vi "Calibrate.vi"(0 "CART TCP Connection In":refnum<k5>, 7 "Calibrate Config":T1={"Frequency, MHz"=2412, "TX Gain"=0, "Data Rate"="1,0,0", "Packet Length"=4, "Packet Count"=4}, 11 "error in (no error)":errorcluster) -> (4 "CART TCP Connection Out":refnum<k5>, 6 "Messages Logged":string[](array[string]), 14 "Command Sent":string, 15 "error out":errorcluster)   [LabVIEW 2011, in "ART2 Test Panel.lvlib"]
uses:
  ART2 Test Panel.lvlib
  Controls/Calibrate Config.ctl
  CART/Controls/Data Rates.ctl
  Controls/Calibrate TXP modes.ctl
  CART/Controls/Inter Frame Spacing modes.ctl
  CART/Controls/Parameter.ctl
  SubVIs/NART Constants.vi
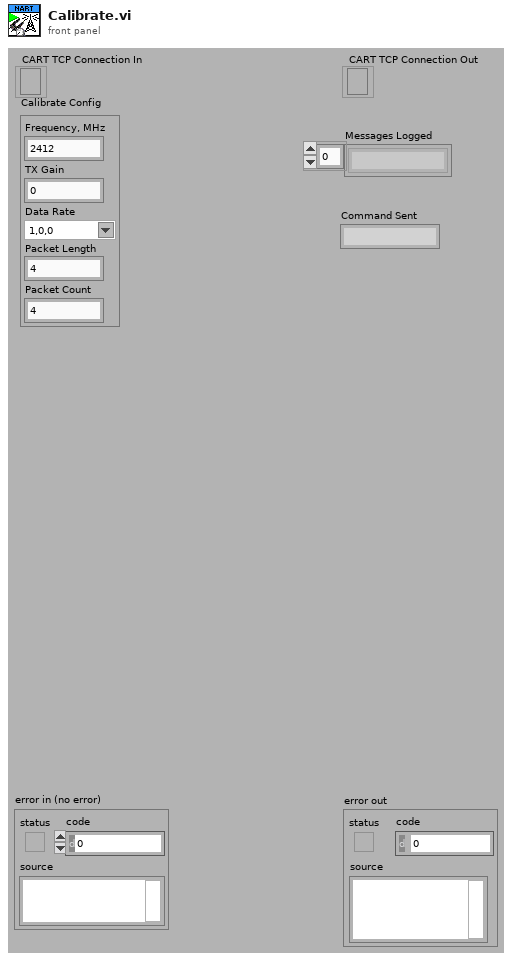
[diagram p1: front panel]
types:
  T1 = typedef "ART2 Test Panel.lvlib/Calibrate Config.ctl" = cluster{"Frequency, MHz":u32, "TX Gain":u32, "Data Rate":T2, "Packet Length":u32, "Packet Count":i32}
  T2 = typedef "ART2 Test Panel.lvlib/Data Rates.ctl" = string
  T3 = typedef "Calibrate TXP modes.ctl" = enum16{"none", "combined", "isolated", "iterate-combined ", "iterate-isolated"}
  T4 = typedef "ART2 Test Panel.lvlib/Parameter.ctl" = cluster{"Name":string, "Type":enum16{"decimal", "string", "float", "hex"}}
  T5 = typedef "ART2 Test Panel.lvlib/Inter Frame Spacing modes.ctl" = i16
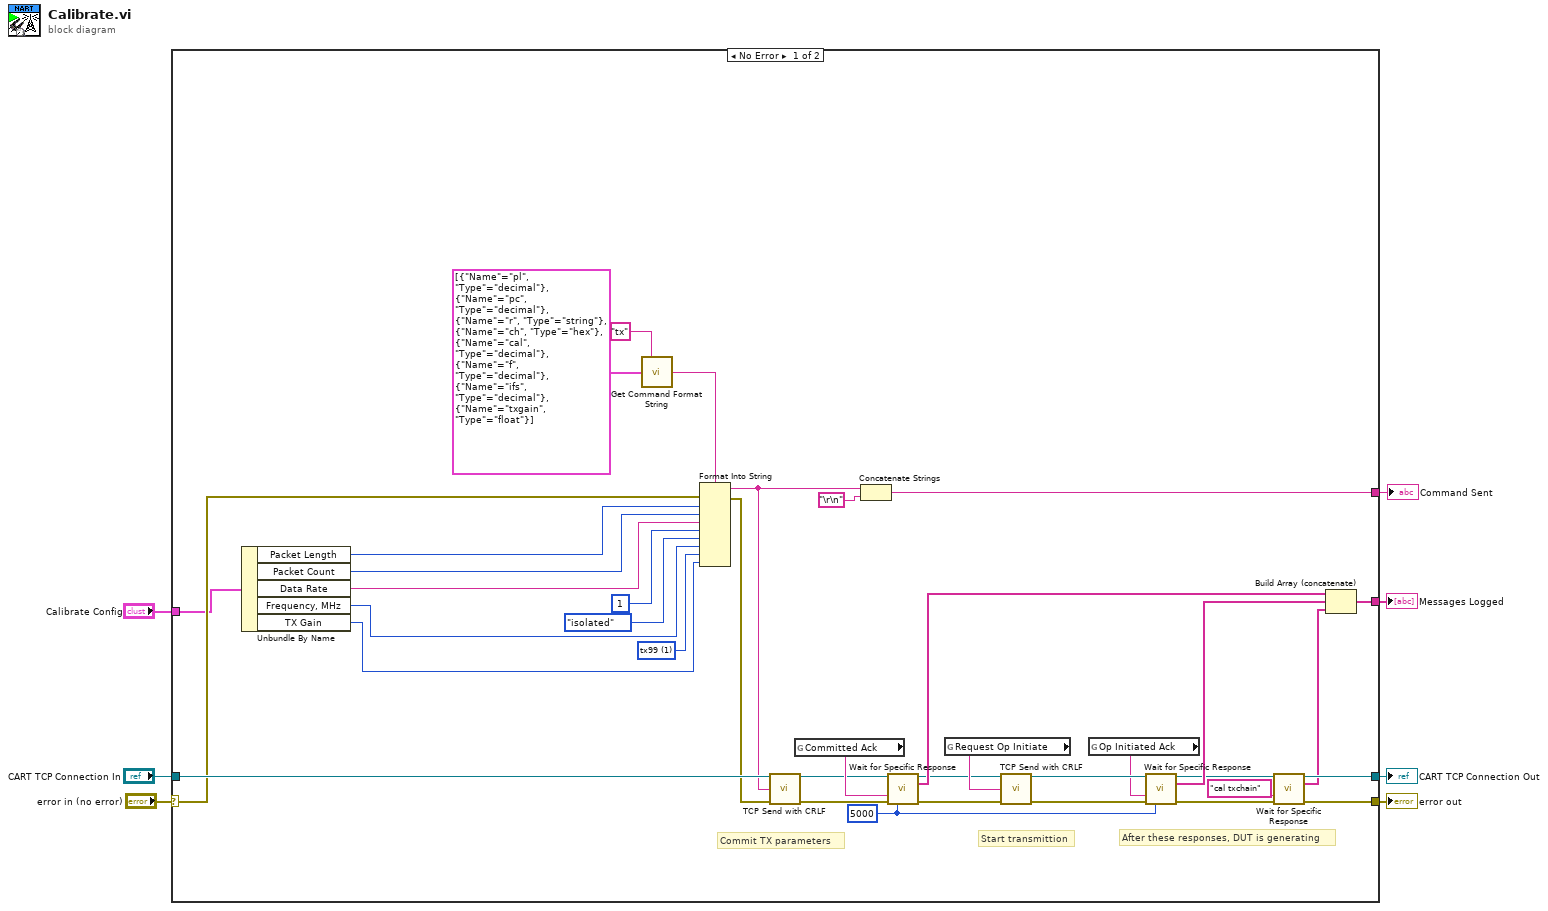
[diagram p0: block diagram]
diagram:
  n1 = case shown="No Error" "error in (no error)" {
    selector: "error in (no error)" -> [w43 w46]
    tunnel: [w9 w46] -> w6
    tunnel: "CART TCP Connection In" -> [w44 w45]
    tunnel: [w10 w45] -> w4
    tunnel: "Calibrate Config" -> [w41 _]
    tunnel: [w36 _] -> w2
    tunnel: [w19 _] -> w1
    frame No Error {
      w16 = T5 1 items=["Regular"=-1, "tx100"=0, "tx99"=1] ("Inter Frame Spacing")
      w39 = 5000 ("Timeout (100ms)")
      # "Start transmittion"
      # "After these responses, DUT is generating"
      # "Commit TX parameters"
      n2 = Unbundle By Name(w41) -> ("Packet Length"=w40:u32, "Packet Count"=w26:i32, "Data Rate"=w17:T2, "Frequency, MHz"=w23:u32, "TX Gain"=w21:u32)
      n3 = call "Get Command Format String.vi"("Command"="tx", "Parameters"=T4[] [{"Name"="pl", "Type"=enum."decimal"}, {"Name"="pc", "Type"=enum."decimal"}, {"Name"="r", "Type"=enum."string"}, {"Name"="ch", "Type"=enum."hex"}, {"Name"="cal", "Type"=enum."decimal"}, {"Name"="f", "Type"=enum."decimal"}, {"Name"="ifs", "Type"=enum."decimal"}, {"Name"="txgain", "Type"=enum."float"}]) -> ("Command Format String"=w22:string)  [unwired: 13 in]
      n4 = Format Into String(format string=w22, error in=w43, w40, w26, w17, u32 1 ("Chains"), Calibrate_TXP_modes."isolated" ("Calibrate TXP"), w23, w16, w21) -> (resulting string=w20:string, error out=w42:errorcluster)  [unwired: 1 in]
      n5 = call "TCP Send with CRLF.vi"("CART TCP Connection"=w44, "data in"=w20, "error IO"=w42) -> ("CART TCP Connection Out"=w34:refnum<k5>, "error out"=w33:errorcluster)  [unwired: 11 in]
      n6 = global read "NART Constants.vi" "Committed Ack"() -> (w35:string)
      n7 = Concatenate Strings(w20, "\r\n") -> (w19:string)
      n8 = call "Wait for Specific Response.vi"("TCP Connection In"=w34, "Expected Message Start (\"\":any)"=w35, "error in"=w33, "Timeout (250 ms)"=w39) -> ("TCP Connection Out"=w30:refnum<k5>, "TCP Messages"=w38:string[], "error out"=w31:errorcluster)  [unwired: 8 in, 1 out]
      n9 = global read "NART Constants.vi" "Request Op Initiate"() -> (w32:string)
      n10 = call "TCP Send with CRLF.vi"("CART TCP Connection"=w30, "data in"=w32, "error IO"=w31) -> ("CART TCP Connection Out"=w29:refnum<k5>, "error out"=w27:errorcluster)  [unwired: 11 in]
      n11 = global read "NART Constants.vi" "Op Initiated Ack"() -> (w28:string)
      n12 = call "Wait for Specific Response.vi"("TCP Connection In"=w29, "Expected Message Start (\"\":any)"=w28, "error in"=w27, "Timeout (250 ms)"=w39) -> ("TCP Connection Out"=w12:refnum<k5>, "TCP Messages"=w37:string[], "error out"=w13:errorcluster)  [unwired: 8 in, 1 out]
      n13 = call "Wait for Specific Response.vi"("TCP Connection In"=w12, "Expected Message Start (\"\":any)"="cal txchain" ("Expected Message Start (\"\":any)"), "error in"=w13) -> ("TCP Connection Out"=w10:refnum<k5>, "TCP Messages"=w8:string[], "error out"=w9:errorcluster)  [unwired: 9 in, 1 out]
      n14 = Build Array (concatenate)(w38, w37, w8) -> (w36:string[])
    }
    frame Error {
    }
  }
  "error out" <- w6
  "CART TCP Connection Out" <- w4
  "Messages Logged" <- w2
  "Command Sent" <- w1
